vi "SEA_TORQUE_CONTROL_PI_CURRENT_CONTROL_REFERENCE.vi"() -> ()   [LabVIEW 2019]
uses:
  Torque control target data.ctl
  <vilib>/Platform/TimedLoop/XDataNode/timing_clust.ctl
  <vilib>/Platform/TimedLoop/XDataNode/nitl_modes.ctl
  <vilib>/Platform/TimedLoop/XDataNode/wakeup.ctl
  <vilib>/FPGAPlugInAG/sbRIO-9627/niLvFpga_Open_sbRIO-9627.vi
  <vilib>/rvi/interface/common/dynamic/niFpgaDynamicAddResources.vi
  <vilib>/Utility/error.llb/Error Cluster From Error Code.vi
  <vilib>/rvi/errors/niLvFpgaAdjustHostInterfaceError.vi
  <vilib>/FPGAPlugInAG/Dynamic/niLvFpga_Close_Dynamic.vi
  <vilib>/rvi/interface/nirviOpenFPGA/nirviOpenFPGA.xnode
  FPGA Bitfiles/seafinalexperime_FPGATarget_SEALOWERLEVELPIC_AplcQzvwIw0.lvbitx
  SEA_LOWER_LEVEL_PI_CONTROL.vi
  <vilib>/platform/TimedLoop/XDataNode/XDataNode.xnode
  <vilib>/rvi/interface/nirviReadWriteControl/nirviReadWriteControl.xnode
  <vilib>/rvi/interface/nirviCloseFPGA/nirviCloseFPGA.xnode
  <vilib>/Platform/TimedLoop/XDataNode/XDNodeRunTimeDep.lvlib
  NiFpgaLv.dll
  <vilib>/rvi/interface/Simulation/niFpgaSimulationCallBeginRW.vi
panel:
  out "Finished late count":u32
  in  "Cluster":T1
  out "Current":cluster{sgl, "filtered current":sgl}(graph)
  out "Torque":cluster{sgl, sgl}(graph)
  in  "Lower limit":sgl
  in  "Upper limit":sgl
  in  "Ki torque":sgl
  in  "Kp torque":sgl
  in  "Amplitude":sgl
  in  "frequency":sgl
  in  "Position Reset":bool
  in  "Position Reset joint side":bool
  in  "Lower bound":sgl
  in  "Upper bound":sgl
  in  "Ki current control":sgl
  in  "Kp current control":sgl
  in  "Current Offset":sgl
  in  "stop":bool
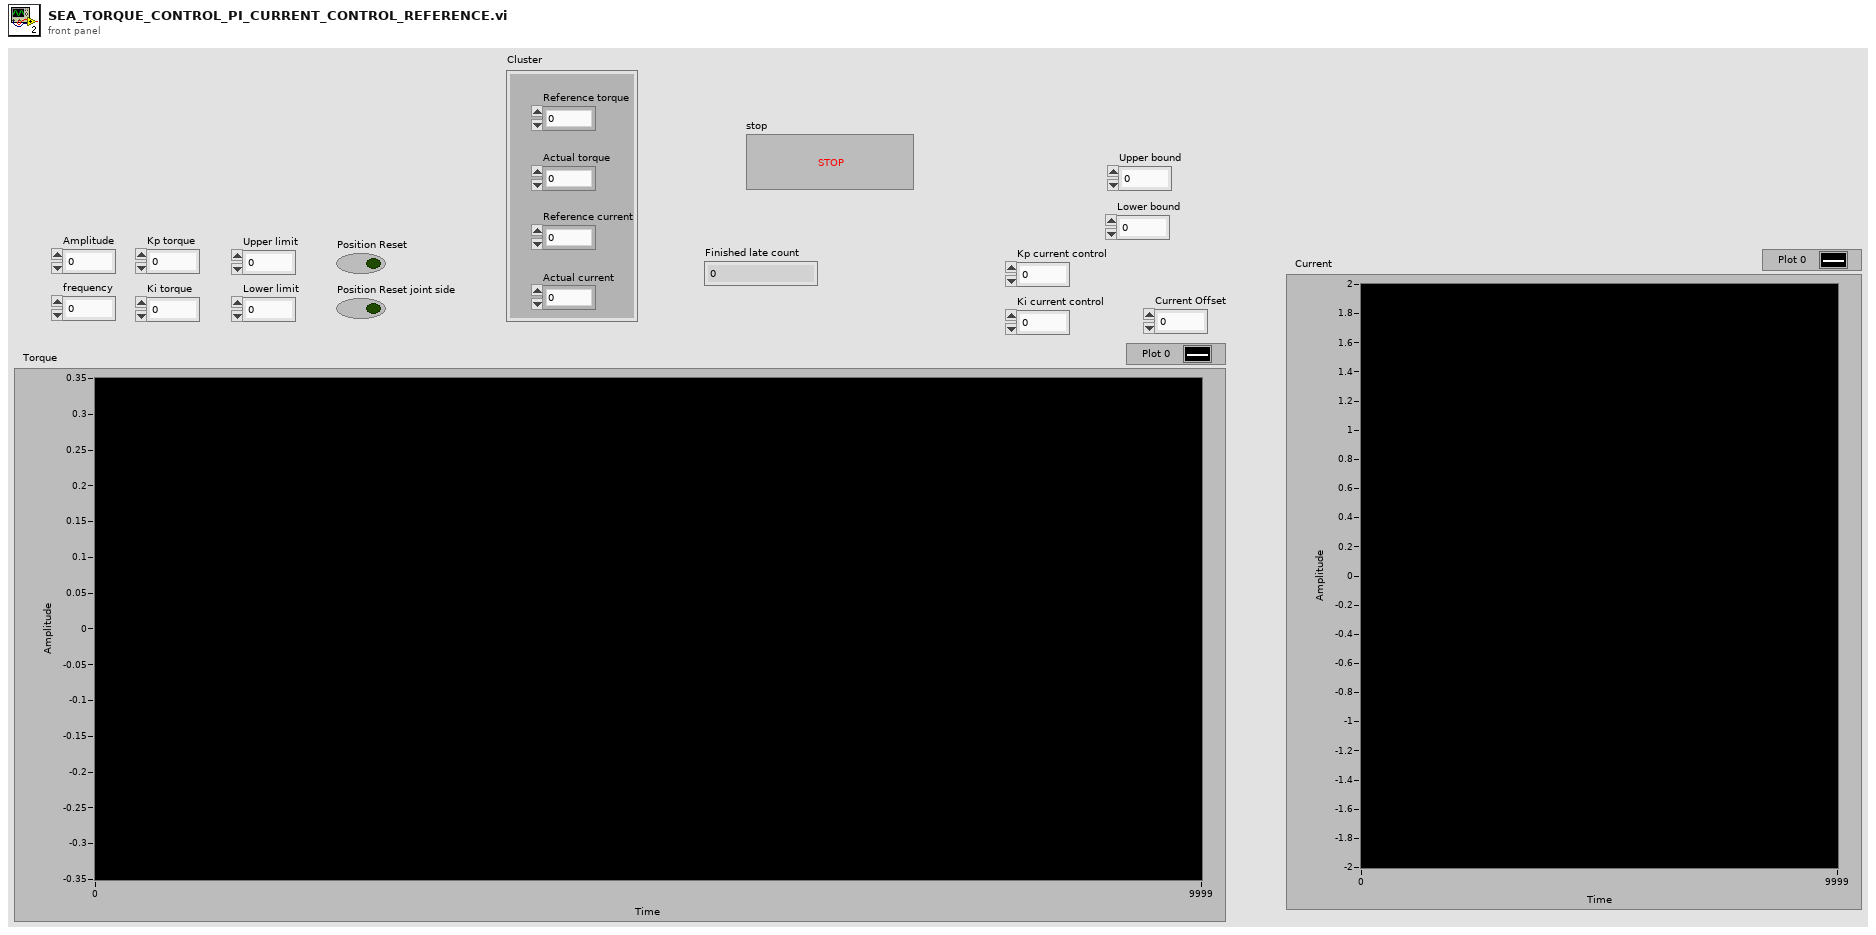
[diagram p1: front panel]
types:
  T1 = typedef "Torque control target data.ctl" = cluster{"Reference torque":sgl, "Actual torque":sgl, "Reference current":sgl, "Actual current":sgl}
  T2 = typedef "XDNodeRunTimeDep.lvlib/timing_clust.ctl" = cluster{"Expected End [f-1]":u64, "Actual End [f-1]":u64, "Finished Late? [f-1]":bool, "Expected End [i-1]":u64, "Actual End [i-1]":u64, "Finished Late? [i-1]":bool, "Expected Start [i]":u64, "Actual Start [i]":u64, "Expected Start [f]":u64, "Actual Start [f]":u64, "Source Name":string, "Structure Name":string, "Period":i64, "Deadline":i64, "Offset":i64, "Start":i64, "Priority":i32, "Timeout":i32, "Mode":T3, "Wakeup Reason":T4, "Error":errorcluster, "Source Type":string, "Secondary Source Type":string, "Global End Time":u64, "Global Start Time":u64, "Frame Duration":u64, "Iteration Duration":u64, "Assigned CPU":i32, "I/O Scan Engine Mode":u32}
  T3 = typedef "XDNodeRunTimeDep.lvlib/nitl_modes.ctl" = enum32{"No Change", "Process missed periods, maintain original phase", "Discard missed periods, maintain original phase", "Process missed periods, ignore original phase", "Discard missed periods, ignore original phase"}
  T4 = typedef "XDNodeRunTimeDep.lvlib/wakeup.ctl" = enum32{"Normal", "Aborted", "Asynchronous wakeup", "Timing source error", "Timed loop error", "Timeout"}
  T5 = enum16{"open", "open or create", "create or replace", "create", "open (read-only)"}
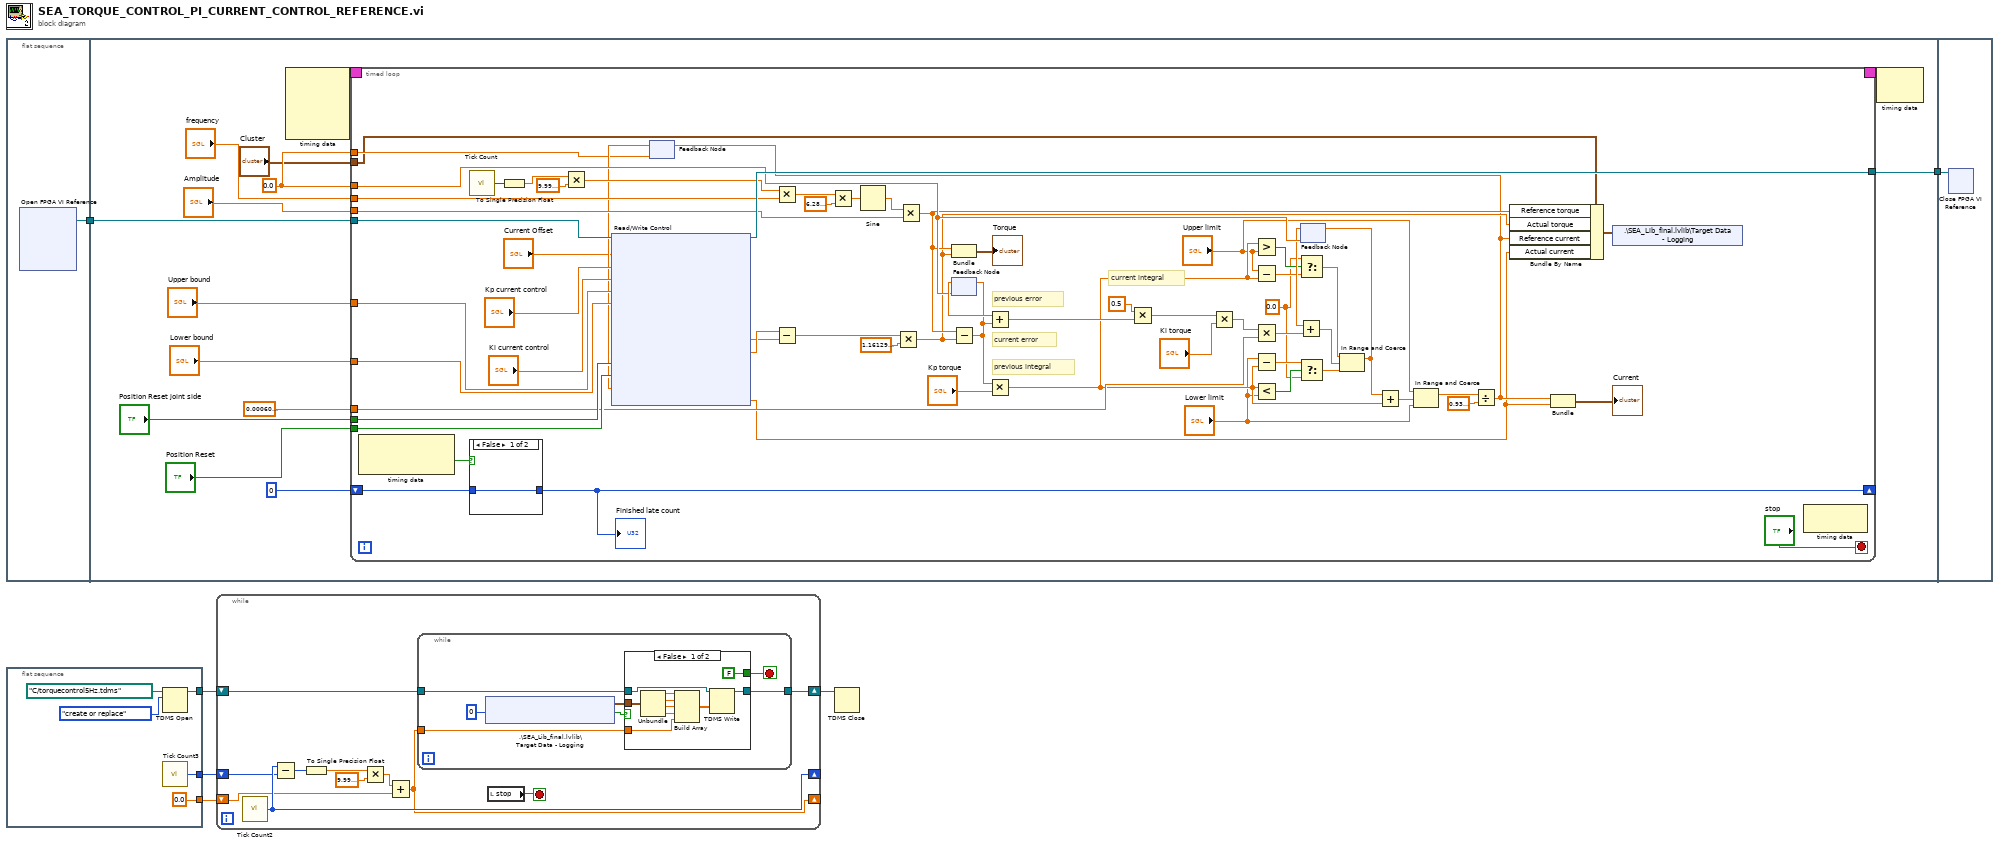
[diagram p0: block diagram]
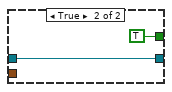
[diagram p2: hidden frame]
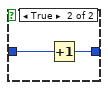
[diagram p3: hidden frame]
diagram:
  n1 = flat-sequence {
    tunnel: [w7] -> w2
    tunnel: w2 -> [w19]
    tunnel: [w18] -> w1
    tunnel: w1 -> [w94]
    frame #0 {
      n2 = xnode "Open FPGA VI Reference"() -> ("FPGA VI Reference Out"=w7:refnum<k20>)  [unwired: 2 in, 1 out]
    }
    frame #1 {
      w9 = sgl 0.0
      n3 = node-c288() -> (w21:T2)  [unwired: 4 in]
      n4 = timed-loop {
        timing: w21 -> [_]
        timing-out: [_] -> w20
        tunnel: w19 -> [w84]
        tunnel: [w83] -> w18
        shift-right: [w80] -> _
        shift-left: u32 0 -> [w81]
        tunnel: "Upper bound" -> [w77]
        tunnel: "Lower bound" -> [w76]
        tunnel: "Position Reset joint side" -> [w75]
        tunnel: "Position Reset" -> [w74]
        tunnel: "frequency" -> [w66]
        tunnel: "Amplitude" -> [w64]
        tunnel: w9 -> [w50]
        tunnel: sgl 0.0006 ("y") -> [w51]
        tunnel: w9 -> [w31]
        tunnel: "Cluster" -> [w28]
        stop <- "stop" stop-if-true
        w43 = sgl 0.0 ("t")
        # "previous integral"
        # "current integral"
        # "previous error"
        # "current error"
        n5 = node-c288() -> (w82:bool)  [unwired: 1 in, 1 out]
        n6 = call "Tick Count"() -> ("Tick Count(uSec)"=w70:u32)
        n7 = case shown="False" w82 {
          tunnel: w81 -> [w86 w88]
          tunnel: [w86 w87] -> w80
          frame False {
          }
          frame True {
            n8 = Increment(x=w88) -> (x+1=w87:u32)
          }
        }
        "Finished late count" <- w80
        n9 = To Single Precision Float(number=w70) -> (single precision float=w69:sgl)
        n10 = Multiply(x=w69, y=sgl 1e-06) -> (x*y=w67:sgl)
        n11 = feedback #1(w31) -> (w32:sgl)
        n12 = xnode "Read/Write Control"("FPGA VI Reference In"=w84, "Current Offset"="Current Offset", "Kp current control"="Kp current control", "Ki current control"="Ki current control", "Upper bound"=w77, "Lower bound"=w76, "Position Reset joint side"=w75, "Position Reset"=w74, "Reference"=w32) -> ("FPGA VI Reference Out"=w83:refnum<k20>, "Position(Radians) joint side"=w62:sgl, "Position(Radians) motor side"=w63:sgl, "filtered current"=w24:sgl)  [unwired: 1 in, 3 out]
        n13 = Multiply(x=w67, y=w66) -> (x*y=w65:sgl)
        n14 = Subtract(x=w63, y=w62) -> (x-y=w61:sgl)
        n15 = Multiply(x=w65, y=sgl 6.28) -> (x*y=w73:sgl)
        n16 = Sine(x=w73) -> (sin(x)=w72:sgl)
        n17 = Multiply(x=w61, y=sgl 1.1613) -> (x*y=w26:sgl)
        n18 = Multiply(x=w72, y=w64) -> (x*y=w27:sgl)
        n19 = Bundle(w27, w26) -> (→"Torque":cluster{sgl, sgl})  [unwired: 1 in]
        n20 = feedback #2(w50) -> (w58:sgl)
        n21 = Subtract(x=w27, y=w26) -> (x-y=w57:sgl)
        n22 = feedback-in #2(w57) -> ()
        n23 = Add(x=w58, y=w57) -> (x+y=w56:sgl)
        n24 = Multiply(x=w57, y="Kp torque") -> (x*y=w38:sgl)
        n25 = Multiply(x=sgl 0.5, y=w56) -> (x*y=w54:sgl)
        n26 = Multiply(x=w54, y="Ki torque") -> (x*y=w52:sgl)
        n27 = Greater?(x=w38, y="Upper limit") -> (0:w47:bool)
        n28 = Subtract(x="Upper limit", y=w38) -> (x-y=w46:sgl)
        n29 = Multiply(x=w52, y=w51) -> (x*y=w49:sgl)
        n30 = Subtract(x="Lower limit", y=w38) -> (x-y=w44:sgl)
        n31 = Less?(x=w38, y="Lower limit") -> (x < y?=w45:bool)
        n32 = Select(t=w43, s=w47, f=w46) -> (s? t:f=w41:sgl)
        n33 = Select(t=w44, s=w45, f=w43) -> (s? t:f=w40:sgl)
        n34 = feedback #3(w50) -> (w48:sgl)
        n35 = Add(x=w48, y=w49) -> (x+y=w42:sgl)
        n36 = In Range and Coerce(upper limit=w41, x=w42, lower limit=w40) -> (coerced(x)=w39:sgl)  [unwired: 1 out]
        n37 = feedback-in #3(w39) -> ()
        n38 = Add(x=w39, y=w38) -> (x+y=w37:sgl)
        n39 = In Range and Coerce(upper limit="Upper limit", x=w37, lower limit="Lower limit") -> (coerced(x)=w34:sgl)  [unwired: 1 out]
        n40 = Divide(x=w34, y=sgl 0.94) -> (x/y=w25:sgl)
        n41 = feedback-in #1(w25) -> ()
        n42 = Bundle By Name(cluster=w28, "Reference torque"=w27, "Actual torque"=w26, "Reference current"=w25, "Actual current"=w24) -> (w23:T1)
        n43 = Bundle(w25, "filtered current"=w24) -> (→"Current":cluster{sgl, "filtered current":sgl})  [unwired: 1 in]
        n44 = shared-variable ".\\SEA_Lib_final.lvlib\\Target Data - Logging"(w23) -> ()  [unwired: 1 in, 1 out]
        n45 = node-c288() -> ()  [unwired: 1 in, 1 out]
      }
      n46 = node-c288(w20) -> ()  [unwired: 1 out]
    }
    frame #2 {
      n47 = xnode "Close FPGA VI Reference"("FPGA VI Reference In"=w94) -> ()  [unwired: 1 in, 1 out]
    }
  }
  n48 = flat-sequence {
    tunnel: [w97] -> w6
    tunnel: [w96] -> w4
    tunnel: [sgl 0.0] -> w3
    frame #0 {
      n49 = TDMS Open(10:T5."create or replace" ("operation (0:open)"), 11:path "C:/torquecontrol5Hz.tdms" ("file path")) -> (3:w97:refnum<k34>)  [unwired: 5 in, 1 out]
      n50 = call "Tick Count3"() -> ("Tick Count(uSec)"=w96:u32)
    }
  }
  n51 = while {
    shift-right: [w109] -> w5
    shift-left: w6 -> [w110]
    shift-right: [w108] -> _
    shift-left: w4 -> [w107]
    shift-right: [w101] -> _
    shift-left: w3 -> [w102]
    stop <- w100 stop-if-true
    n52 = call "Tick Count2"() -> ("Tick Count(uSec)"=w108:u32)
    n53 = Subtract(x=w108, y=w107) -> (x-y=w106:u32)
    n54 = To Single Precision Float(number=w106) -> (single precision float=w105:sgl)
    n55 = Multiply(x=w105, y=sgl 1e-06) -> (x*y=w104:sgl)
    n56 = Add(x=w104, y=w102) -> (x+y=w101:sgl)
    n57 = while {
      tunnel: w110 -> [w114]
      tunnel: [w112] -> w109
      tunnel: w101 -> [w111]
      stop <- w115 stop-if-true
      n58 = shared-variable ".\\SEA_Lib_final.lvlib\\Target Data - Logging"(0 ("ms timeout (0)")) -> (w113:T1, w116:bool)  [unwired: 1 in, 1 out]
      n59 = case shown="False" w116 {
        tunnel: [FALSE TRUE] -> w115
        tunnel: w114 -> [w127 w128]
        tunnel: w113 -> [w126 _]
        tunnel: [w120 w128] -> w112
        tunnel: w111 -> [w118 _]
        frame False {
          n60 = Unbundle(w126) -> ("Reference torque"=w125:sgl, "Actual torque"=w124:sgl, "Reference current"=w123:sgl, "Actual current"=w122:sgl)
          n61 = Build Array(w125, w124, w123, w122, w118) -> (w121:sgl[])
          n62 = TDMS Write(0:w127, 9:w121) -> (4:w120:refnum<k34>)  [unwired: 4 in, 3 out]
        }
        frame True {
        }
      }
    }
    n63 = local read "stop"() -> (w100:bool)
  }
  n64 = TDMS Close(11:w5) -> ()  [unwired: 1 in, 2 out]
